vi "Topo & GridSpectr_DriftCorrection_v4.vi"(6 "Internal use":string, 7 "Grid param":T2 {"height (m)" format="%#_6p"; "width (m)" format="%#_6p"; "center Y (m)" format="%#_6p"; "center X (m)" format="%#_6p"}, 8 "Error in (no error)":errorcluster, 9 "Points Y/Index Y":i32, 10 "Points X/Index X":i32, 11 "Method":enum16{"init", "run", "end"}(ring)=enum."end") -> (0 "Error out":errorcluster)   [LabVIEW 2014]
doc: "Example of a measurement VI to be used in the \"Experiments on a Grid\" tool as external VI.\n\nThis example measure the topography and spectroscopy data. The spectroscopy measurements are taken on a subgrid. The data are saved to a sxm and a binary file.\n\n- Nanonis Programming Interface -"
uses:
  <userlib>/Nanonis Prog Interface V5/Nanonis Prog Interface.lvlib
panel:
  in  "STS current step":dbl format="%#_6p"
  in  "tip Speed (m/s)":sgl=3e-09 format="%.2p"
  in  "Drift Correction 2":T1
  out "X drift":i32
  out "Y drift":i32
  out "Queue Steps":i32=40
  in  "StepsBack":i32=40
  in  "Channel index (0-23)":u8=14
  in  "File name":string="10_mol_chain"
  in  "STS Current":dbl=1e-11 format="%#_6p"
  in  "Imaging Current":dbl=1e-10 format="%#_6p"
  in  "zdrift \nDuration (s)":dbl
  in  "Correct z drift":bool
  out "Status":string="init"
  in  "Drift correction Pixels":i32=256 caption="Pixels for drift correction"
  out "Y Offset":dbl
  out "X Offset":dbl
  out "Points taken":dbl
  in  "Drift Correction every":i32=34
  in  "Y subgrid spacing":u16=1
  in  "X subgrid spacing":u16=1
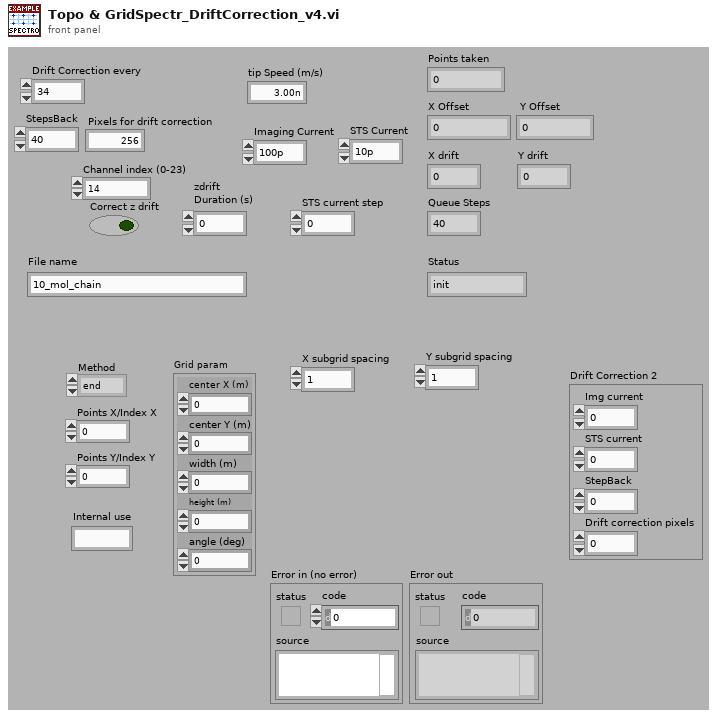
[diagram p1: front panel]
types:
  T1 = cluster{"Img current":dbl, "STS current":dbl, "StepBack":dbl, "Drift correction pixels":dbl}
  T2 = cluster{"center X (m)":sgl, "center Y (m)":sgl, "width (m)":sgl, "height (m)":sgl, "angle (deg)":sgl}
  T3 = cluster{"center X":sgl, "center Y":sgl, "angle":sgl, "width":sgl, "height":sgl, "# pixels":i32, "# lines":i32}
  T4 = cluster{"Name":string, "Calibration":sgl, "Offset":sgl, "Channel index":i32}[]
  T5 = cluster{"up/down":bool, "time/line":sgl, "start time":timestamp, "end time":timestamp}
  T6 = cluster{"Z averaging time (s)":sgl, "Z offset (m)":sgl, "Initial settling time (s)":sgl}
  T7 = cluster{"Max. slew rate (V/s)":sgl, "Settling time (s)":sgl, "Integration time (s)":sgl}
  T8 = cluster{"End settling time (s)":sgl, "Z control time (s)":sgl}
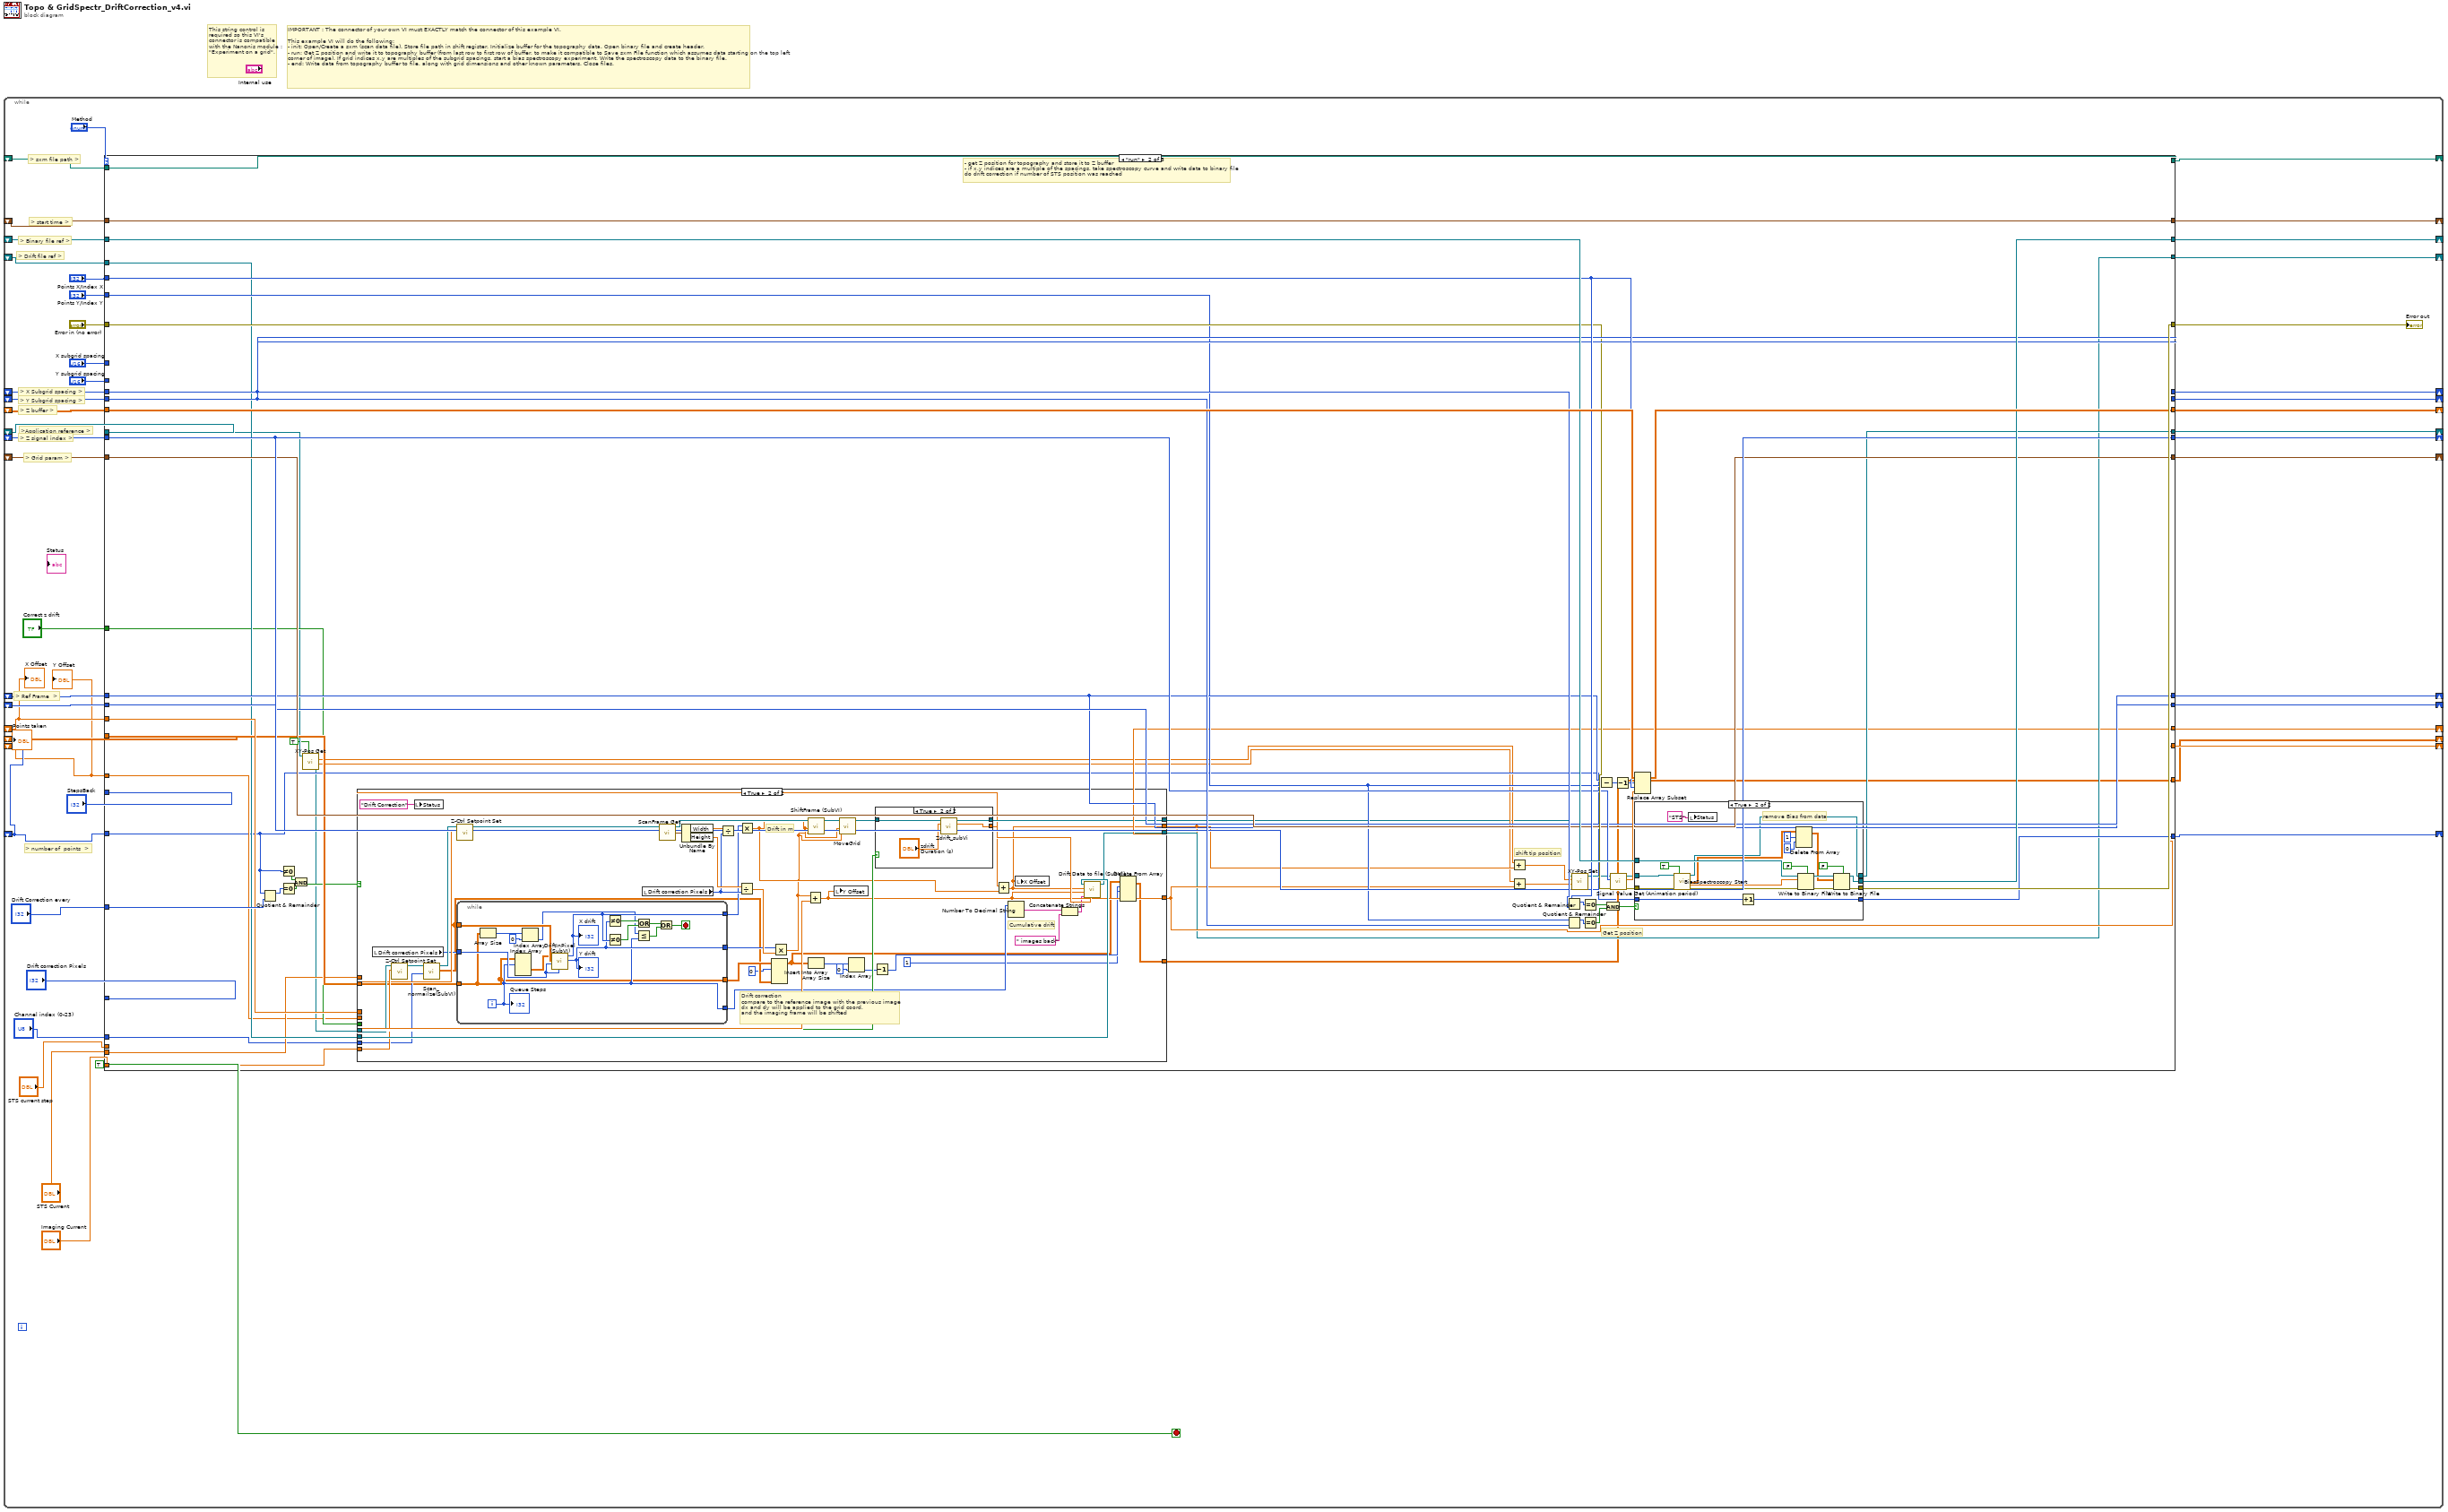
[diagram p0: block diagram]
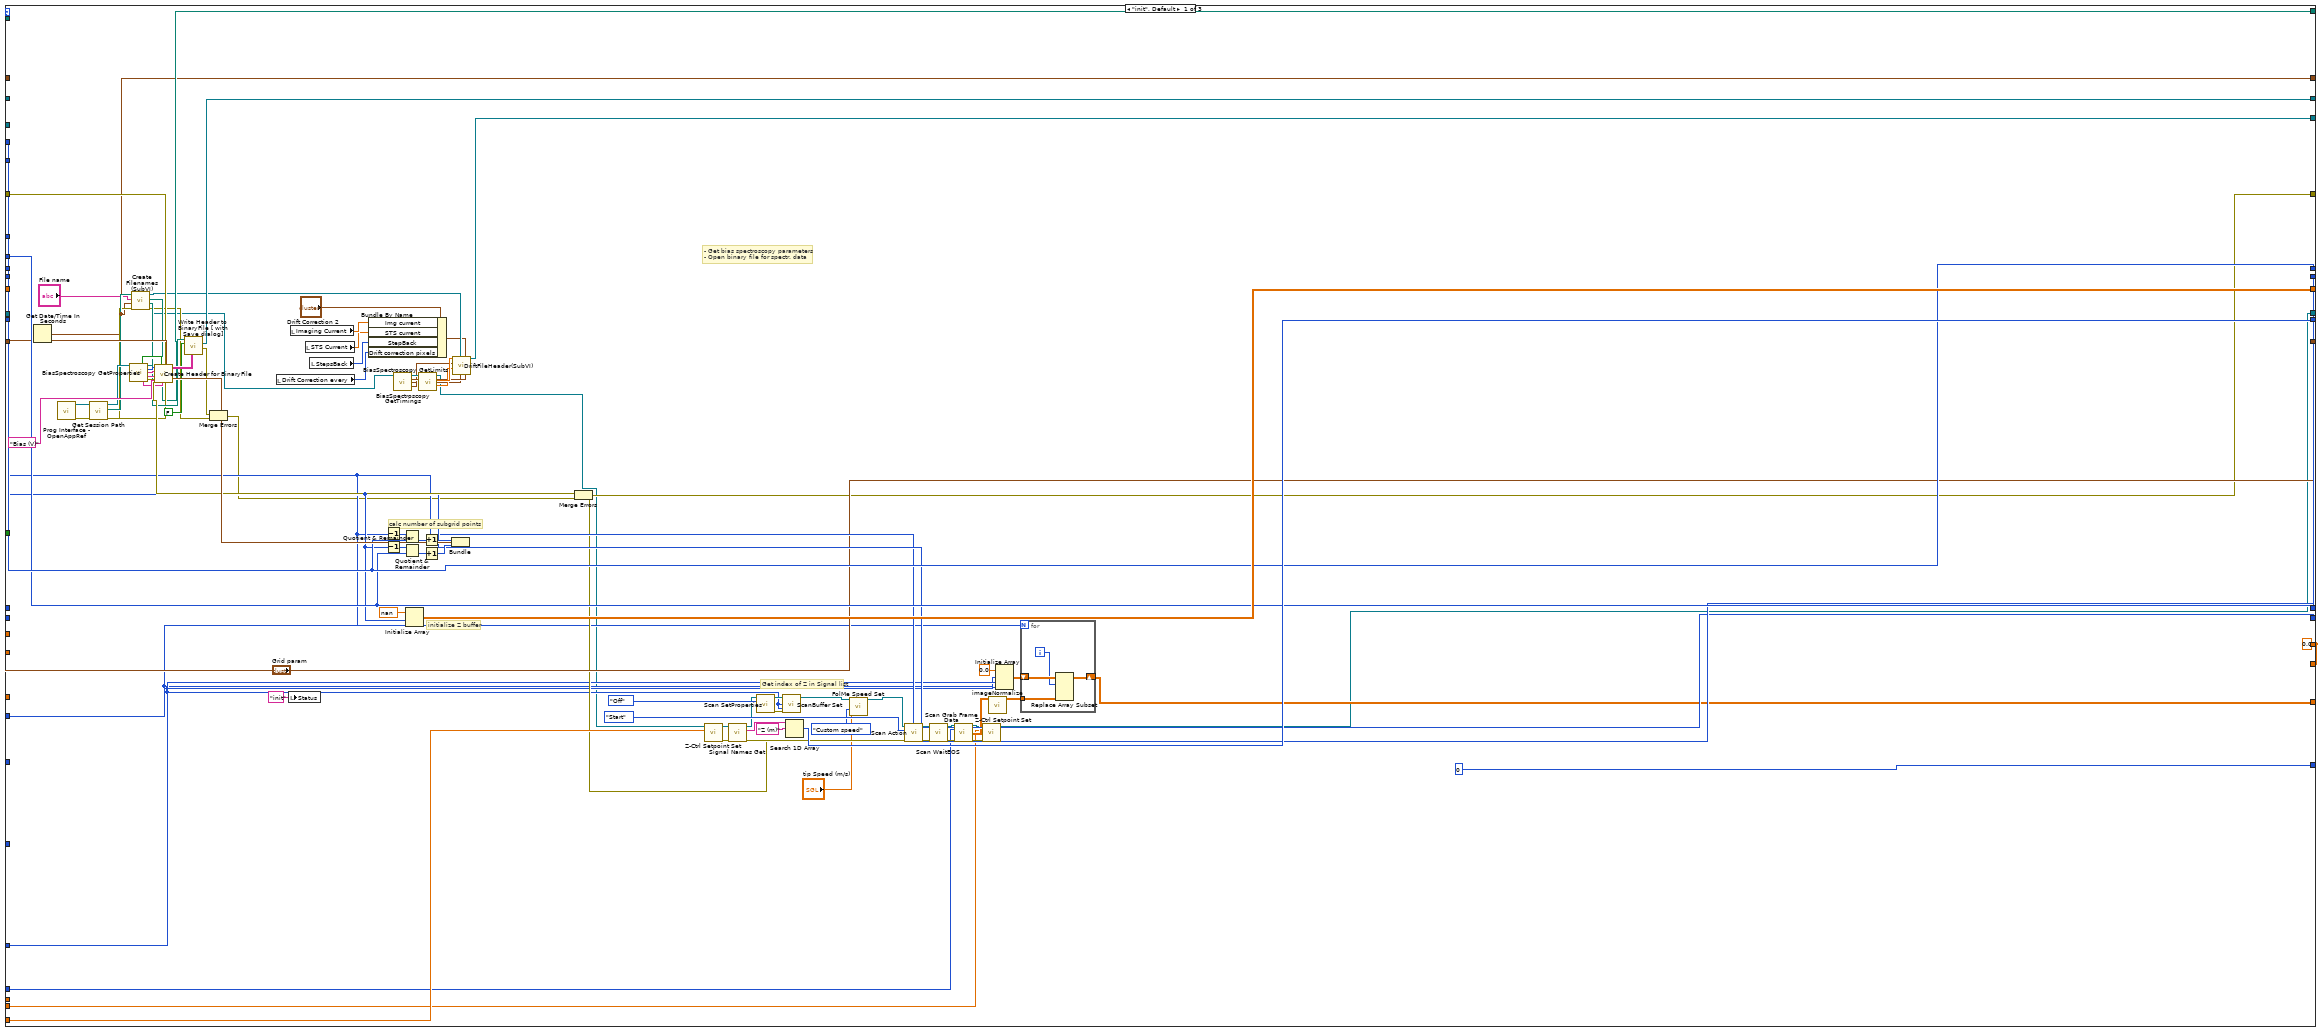
[diagram p2: hidden frame]
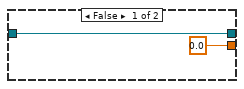
[diagram p4: hidden frame]
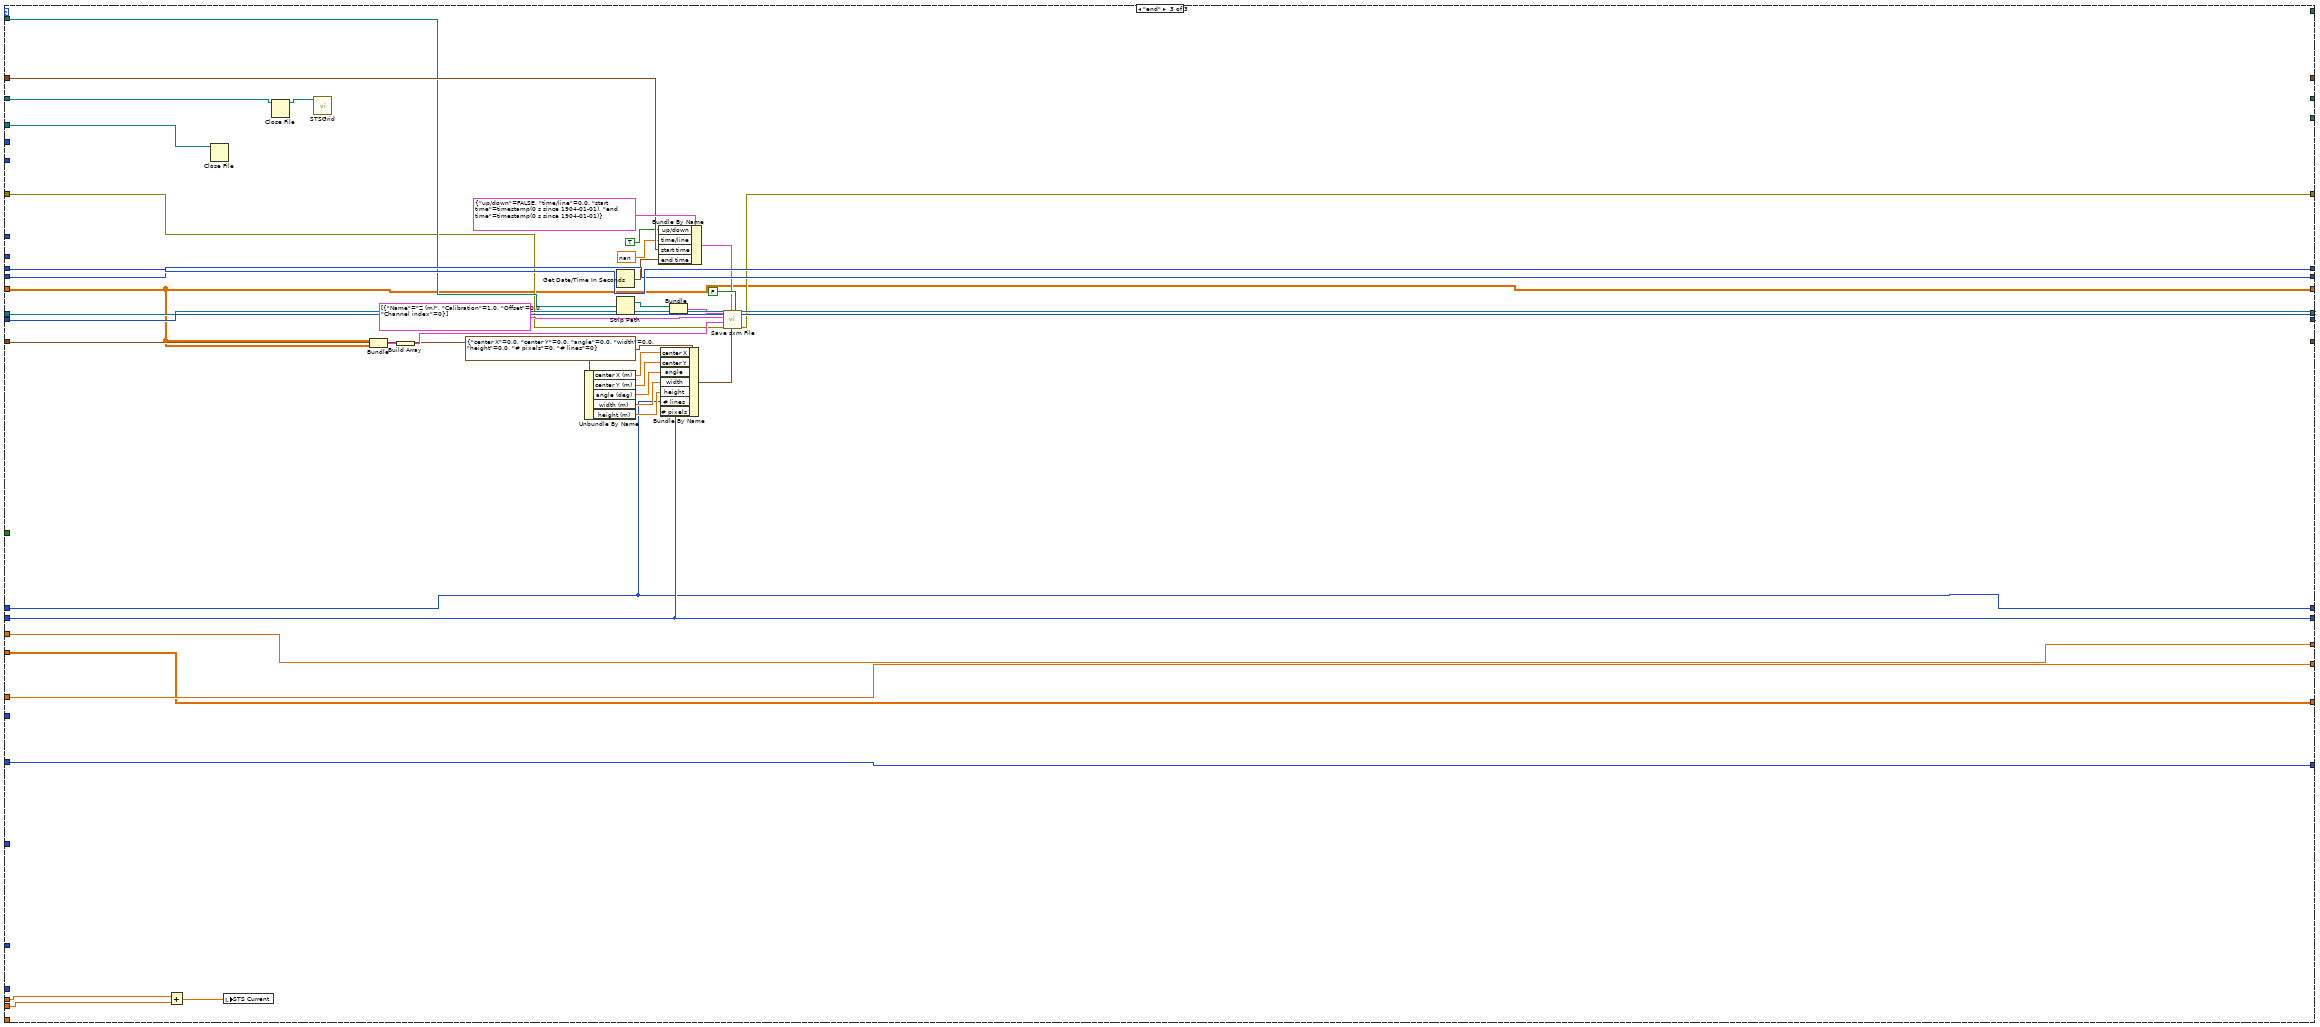
[diagram p6: hidden frame]
diagram:
  # "This string control is required so this VI's connector is compatible with the Nanonis module : \"Experiment on a grid\"."
  # "IMPORTANT : The connector of your own VI must EXACTLY match the connector of this example VI.\n\nThis example VI will do the following:\n- init: Open/Create a sxm (scan data file). Store file path in shift register. Initialize buffer for the topography data. Open binary file and create header.\n- run: Get Z position and write it to topography buffer (from last row to first row of buffer, to make it compatible to Save sxm File function which assumes data starting on the top left corner of image). If grid indices x,y are multiples of the subgrid spacings, start a bias spectroscopy experiment. Write the spectroscopy data to the binary file.\n- end: Write data from topography buffer to file, along with grid dimensions and other known parameters. Close files."
  n1 = while {
    shift-right: [w23] -> _
    shift-left: _ -> [w46]
    shift-right: [w41] -> _
    shift-left: _ -> [w40]
    shift-right: [w38] -> _
    shift-left: _ -> [w39]
    shift-right: [w37] -> _
    shift-left: _ -> [w36]
    shift-right: [w30] -> _
    shift-left: _ -> [w32]
    shift-right: [w31] -> _
    shift-left: _ -> [w33]
    shift-right: [w29] -> _
    shift-left: _ -> [w28]
    shift-right: [w27] -> _
    shift-left: _ -> [w26]
    shift-right: [w25] -> _
    shift-left: _ -> [w24]
    shift-right: [w22] -> _
    shift-left: _ -> [w21]
    shift-right: [w20] -> _
    shift-left: _ -> [w19]
    shift-right: [w18] -> _
    shift-left: _ -> [w11]
    shift-right: [w17] -> _
    shift-left: _ -> [w10]
    shift-right: [w16] -> _
    shift-left: _ -> [w13]
    shift-right: [w15] -> _
    shift-left: _ -> [w12]
    shift-right: [w8] -> _
    shift-left: _ -> [w7]
    stop <- TRUE stop-if-true
    # "> Drift file ref >"
    # "> number of  points  >"
    # "> Ref Frame  >"
    # "> Grid param >"
    # "> start time >"
    # ">Application reference >"
    # "> Y Subgrid spacing >"
    # "> X Subgrid spacing >"
    # "> Z signal index >"
    # "> Binary file ref >"
    # "> Z buffer >"
    # "> sxm file path >"
    n2 = case shown="\"run\"" "Method" {
      tunnel: [w82 w196 _] -> w23
      tunnel: w46 -> [_ w196 w324]
      tunnel: "Error in (no error)" -> [w84 w182 w317]
      tunnel: [w93 w195 w316] -> w44
      tunnel: "Points X/Index X" -> [w113 w190 _]
      tunnel: "Points Y/Index Y" -> [w114 w174 _]
      tunnel: [w137 w193 w305] -> w41
      tunnel: w40 -> [_ w194 w305]
      tunnel: w39 -> [_ w192 w294]
      tunnel: [w129 w191 _] -> w38
      tunnel: [w127 w180 w333] -> w37
      tunnel: w36 -> [_ w180 w333]
      tunnel: "X subgrid spacing" -> [w126 _ _]
      tunnel: "Y subgrid spacing" -> [w125 _ _]
      tunnel: w33 -> [_ w184 w332]
      tunnel: w32 -> [_ w183 w331]
      tunnel: [w126 w184 w332] -> w31
      tunnel: [w125 w183 w331] -> w30
      tunnel: [w55 w166 w330] -> w29
      tunnel: w28 -> [_ w147 w330]
      tunnel: ["Grid param" w177 _] -> w27
      tunnel: w26 -> [_ w177 w315]
      tunnel: [w81 w178 _] -> w25
      tunnel: w24 -> [_ w178 w325]
      tunnel: [w114 w175 w306] -> w22
      tunnel: w21 -> [_ w175 w306]
      tunnel: [w113 w176 w307] -> w20
      tunnel: w19 -> [_ w176 w307]
      tunnel: [w104 w156 w304] -> w18
      tunnel: [w104 w161 w302] -> w17
      tunnel: [w76 w153 w298] -> w16
      tunnel: [0 w171 w303] -> w15
      tunnel: w12 -> [_ w150 w303]
      tunnel: "Drift Correction every" -> [_ w169 _]
      tunnel: w13 -> [_ w160 w298]
      tunnel: w11 -> [_ w167 w304]
      tunnel: w10 -> [_ w151 w302]
      tunnel: "Drift correction Pixels" -> [w75 _ _]
      tunnel: [w71 w158 _] -> w8
      tunnel: w7 -> [_ w159 w299]
      tunnel: "Correct z drift" -> [_ w157 _]
      tunnel: "Imaging Current" -> [w94 w155 _]
      tunnel: "STS Current" -> [w89 w154 w295]
      tunnel: "Channel index (0-23)" -> [w79 w152 _]
      tunnel: "StepsBack" -> [w74 _ _]
      tunnel: "STS current step" -> [_ _ w297]
      frame "init", Default {
        w104 = 0.0
        # "- Get bias spectroscopy parameters\n- Open binary file for spectr. data"
        # "initialize Z buffer"
        # "calc number of subgrid points"
        # "Get index of Z in Signal list"
        n3 = Get Date/Time In Seconds() -> (seconds since 1Jan1904=w81:timestamp)
        n4 = call <userlib>:"Prog Interface - OpenAppRef.vi"("Error in (no error)"=w84) -> ("Error out"=w86:errorcluster, "Application reference"=w88:refnum<vi>)  [unwired: 5 in]
        n5 = call <userlib>:"Get Session Path.vi"("error in (no error)"=w86, "Application ref in"=w88) -> ("error out"=w83:errorcluster, "Session path"=w85:path, "Application ref out"=w87:refnum<vi>)  [unwired: 7 in]
        n6 = call <userlib>:"BiasSpectroscopy GetProperties.vi"("Application ref in"=w87) -> ("Backward sweep"=w133:bool, "Application ref out"=w54:refnum<vi>, "Number of points"=w116:i32, "Channels"=w115:string[], "Parameters"=w131:string[], "Fixed parameters"=w118:string[], "Error out"=w130:errorcluster)  [unwired: 6 in, 2 out]
        n7 = call "Create Filenames (SubVI).vi"("error in (no error)"=w83, "seconds since 1Jan1904"=w81, "File name"="File name", "Session path"=w85) -> ("error out"=w56:errorcluster, "binFilePath"=w97:path, "topoFilePath"=w82:path, "Drift File out"=w72:refnum<file>)  [unwired: 4 in]
        n8 = local read "Drift Correction every"() -> (w66:i32)
        n9 = local write "Status"("init" ("Status")) -> ()
        n10 = local read "Imaging Current"() -> (w68:dbl)
        n11 = local read "STS Current"() -> (w67:dbl)
        n12 = local read "StepsBack"() -> (w65:i32)
        n13 = Bundle By Name(cluster="Drift Correction 2", "Img current"=w68, "STS current"=w67, "StepBack"=w65, "Drift correction pixels"=w66) -> (w69:T1)
        n14 = Decrement(x=w113) -> (x-1=w124:i32)
        n15 = Decrement(x=w114) -> (x-1=w123:i32)
        n16 = call <userlib>:"BiasSpectroscopy GetTimings.vi"("Application ref in"=w54) -> ("Application ref out"=w64:refnum<vi>, "Initialization"=w61:T6, "Sweep Timing"=w59:T7, "End of Sweep"=w60:T8)  [unwired: 10 in, 1 out]
        n17 = Quotient & Remainder(x=w124, y=w126) -> (floor(x/y)=w122:i32)  [unwired: 1 out]
        n18 = Quotient & Remainder(x=w123, y=w125) -> (floor(x/y)=w121:i32)  [unwired: 1 out]
        n19 = Initialize Array(sgl nan ("element"), w114, w113) -> (w137:sgl[][])
        n20 = call <userlib>:"BiasSpectroscopy GetLimits.vi"("Application ref in"=w64) -> ("End value (V)"=w62:sgl, "Start value (V)"=w63:sgl, "Application ref out"=w53:refnum<vi>)  [unwired: 5 in, 1 out]
        n21 = Increment(x=w122) -> (x+1=w120:i32)
        n22 = Increment(x=w121) -> (x+1=w119:i32)
        n23 = Bundle(w120, w119) -> (w132:cluster{i32, i32})  [unwired: 1 in]
        n24 = call <userlib>:"Create Header for BinaryFile.vi"("Grid points"=w132, "Grid param"="Grid param", "Fixed parameters"=w118, "Backward sweep"=w133, "Sweep signal"="Bias (V)" ("Sweep Signal"), "Parameters"=w131, "Channels"=w115, "Points per sweep"=w116) -> ("Header (fixed attributes)"=w135:string[][])  [unwired: 3 in]
        n25 = call <userlib>:"Write Header to BinaryFile [ with Save dialog].vi"("Fixed Attributes"=w135, "Show Dialog? (T)"=FALSE, "Filename"=w97) -> ("Error out"=w57:errorcluster, "File ref"=w129:refnum<file>)  [unwired: 5 in, 2 out]
        n26 = Merge Errors(w57, w56) -> (w58:errorcluster)
        n27 = call "DriftFileHeader(SubVI).vi"("Initialization"=w61, "Drift Correction"=w69, "Sweep Timing"=w59, "Byte Stream File in"=w72, "End value (V)"=w62, "End of Sweep"=w60, "Start value (V)"=w63) -> ("Byte Stream File out"=w71:refnum<file>)  [unwired: 4 in]
        n28 = Merge Errors(w130, w58) -> (w93:errorcluster)
        n29 = call <userlib>:"Z-Ctrl Setpoint Set.vi"("error in (no error)"=w93, "Z Controller setpoint"=w94, "Application ref in"=w53) -> ("error out"=w92:errorcluster, "Application ref out"=w95:refnum<vi>)  [unwired: 7 in]
        n30 = call <userlib>:"Signal Names Get.vi"("error in (no error)"=w92, "Application ref in"=w95) -> ("error out"=w105:errorcluster, "Signals Names"=w117:string[], "Application ref out"=w100:refnum<vi>)  [unwired: 5 in]
        n31 = call <userlib>:"Scan SetProperties.vi"("Application ref in"=w100, "Continuous scan"=enum16{"No change", "On", "Off"}."Off") -> ("Application ref out"=w102:refnum<vi>, "Error out"=w101:errorcluster)  [unwired: 12 in]
        n32 = call <userlib>:"ScanBuffer Set.vi"("Application ref in"=w102, "Pixels"=w75, "Lines"=w75, "error in (no error)"=w101) -> ("Application ref out"=w52:refnum<vi>)  [unwired: 10 in, 1 out]
        n33 = Search 1D Array(1D array=w117, element="Z (m)") -> (index of element=w127:i32)  [unwired: 1 in]
        n34 = call <userlib>:"FolMe Speed Set.vi"("Speed Setting (Custom)"=enum32{"Scan speed", "Custom speed"}."Custom speed", "Speed (m/s)"="tip Speed (m/s)", "Application ref in"=w52) -> ("Application ref out"=w51:refnum<vi>)  [unwired: 5 in, 1 out]
        n35 = call <userlib>:"Scan Action.vi"("error in (no error)"=w105, "Scan action (Start)"=enum16{"Start", "Stop", "Pause", "Resume"}."Start", "Application ref in"=w51) -> ("error out"=w111:errorcluster, "Application ref out"=w110:refnum<vi>)  [unwired: 6 in]
        n36 = call <userlib>:"Scan WaitEOS.vi"("error in (no error)"=w111, "Application ref in"=w110) -> ("error out"=w108:errorcluster, "Application ref out"=w109:refnum<vi>)  [unwired: 5 in, 2 out]
        n37 = call <userlib>:"Scan Grab Frame Data.vi"("Application ref in"=w109, "Channel index (0-23)"=w79, "error in (no error)"=w108) -> ("Application ref out"=w91:refnum<vi>, "Scan frame data"=w96:sgl[][], "error out"=w90:errorcluster)  [unwired: 8 in, 2 out]
        n38 = call <userlib>:"Z-Ctrl Setpoint Set.vi"("error in (no error)"=w90, "Z Controller setpoint"=w89, "Application ref in"=w91) -> ("Application ref out"=w55:refnum<vi>)  [unwired: 7 in, 1 out]
        n39 = call "imageNormalize.vi"("Data"=w96) -> ("Array"=w73:dbl[][])  [unwired: 10 in]
        n40 = Initialize Array(0.0 ("element"), w74, w75, w75) -> (w77:dbl[][][])
        n41 = for {
          N: w74 -> [_]
          tunnel: w73 -> [w140]
          shift-right: [w139] -> w76
          shift-left: w77 -> [w141]
          i -> [w138]
          n42 = Replace Array Subset(array=w141, new element=w140, index (dim 0)=w138) -> (w139:dbl[][][])  [unwired: 2 in]
        }
      }
      frame "run" {
        # "shift tip position"
        # "Get Z position"
        # "- get Z position for topography and store it to Z buffer\n- if x,y indices are a multiple of the spacings, take spectroscopy curve and write data to binary file\ndo drift correction if number of STS position was reached"
        n43 = Quotient & Remainder(x=w150, y=w169) -> (x-y*floor(x/y)=w170:i32)  [unwired: 1 out]
        n44 = Not Equal To 0?(x=w150) -> (x != 0?=w148:bool)
        n45 = Equal To 0?(x=w170) -> (x = 0?=w168:bool)
        n46 = And(x=w148, y=w168) -> (x .and. y?=w149:bool)
        n47 = call <userlib>:"XY-Pos Get.vi"("Wait for newest data (F=False)"=TRUE, "Application ref in"=w147) -> ("Y (m)"=w143:sgl, "X (m)"=w144:sgl, "Application ref out"=w146:refnum<vi>)  [unwired: 5 in, 1 out]
        n48 = case shown="True" w149 {
          tunnel: w146 -> [w201 w232]
          tunnel: [w201 w238] -> w142
          tunnel: w160 -> [w198 w220]
          tunnel: [w200 w234] -> w156
          tunnel: [w199 w233] -> w161
          tunnel: w167 -> [w200 w236]
          tunnel: w151 -> [w199 w237]
          tunnel: [w198 w212] -> w153
          tunnel: w159 -> [w197 w241]
          tunnel: [w197 w240] -> w158
          tunnel: w157 -> [_ w235]
          tunnel: w155 -> [_ w231]
          tunnel: w154 -> [_ w229]
          tunnel: w152 -> [_ w224]
          frame False {
          }
          frame True {
            # "Cumulative drift"
            # "Drift in m"
            # "Drift correction \ncompare to the reference image with the previous image \ndx and dy will be applied to the grid coord, \nand the imaging frame will be shifted"
            n49 = local read "Drift correction Pixels"() -> (w223:i32)
            n50 = call <userlib>:"Z-Ctrl Setpoint Set.vi"("Z Controller setpoint"=w231, "Application ref in"=w232) -> ("Application ref out"=w228:refnum<vi>)  [unwired: 8 in, 1 out]
            n51 = local write "Status"("Drift Correction" ("Status")) -> ()
            n52 = call "Scan_normailze(SubVI).vi"("Channel index (0-23)"=w224, "Application in"=w228) -> ("Array"=w214:dbl[][], "Application out"=w230:refnum<vi>)  [unwired: 7 in, 1 out]
            n53 = call <userlib>:"Z-Ctrl Setpoint Set.vi"("Z Controller setpoint"=w229, "Application ref in"=w230) -> ("Application ref out"=w226:refnum<vi>)  [unwired: 8 in, 1 out]
            n54 = while {
              tunnel: w223 -> [w260]
              tunnel: w214 -> [w259]
              tunnel: w220 -> [w249]
              tunnel: [w258] -> w222
              tunnel: [w257] -> w221
              tunnel: [w253] -> w219
              tunnel: [w249] -> w215
              i -> [w253]
              stop <- w255 stop-if-true
              n55 = Array Size(array=w249) -> (size(s)=w252:i32[])
              n56 = Index Array(array=w249, index (dim 0)=w253) -> (element=w248:dbl[][])  [unwired: 2 in]
              n57 = Index Array(array=w252, index=0) -> (element=w250:i32)
              n58 = call "DriftInPixel (SubVI).vi"(6:w260, 9:w260, "New image"=w259, "Ref image"=w248) -> ("Y drift"=w257:i32, "X drift"=w258:i32)  [unwired: 5 in, 1 out]
              "Y drift" <- w257
              "X drift" <- w258
              n59 = Not Equal To 0?(x=w257) -> (x != 0?=w262:bool)
              n60 = Not Equal To 0?(x=w258) -> (x != 0?=w261:bool)
              n61 = Or(x=w262, y=w261) -> (x .or. y?=w256:bool)
              n62 = Less Or Equal?(x=w250, y=w253) -> (x <= y?=w254:bool)
              n63 = Or(x=w256, y=w254) -> (x .or. y?=w255:bool)
              "Queue Steps" <- w253
            }
            n64 = local read "Drift correction Pixels"() -> (w225:i32)
            n65 = call <userlib>:"ScanFrame Get.vi"("Application ref in"=w226) -> ("Application ref out"=w227:refnum<vi>, "Size (m)"=w246:cluster{"Width":sgl, "Height":sgl})  [unwired: 10 in, 3 out]
            n66 = Unbundle By Name(w246) -> ("Width"=w245:sgl, "Height"=w247:sgl)
            n67 = Divide(x=w245, y=w225) -> (x/y=w244:sgl)
            n68 = Divide(x=w247, y=w225) -> (x/y=w243:sgl)
            n69 = Multiply(x=w222, y=w244) -> (x*y=w203:sgl)
            n70 = Insert Into Array(array=w215, index (dim 0)=0 ("index (page)"), new element=w214) -> (w211:dbl[][][])  [unwired: 2 in]
            n71 = Multiply(x=w221, y=w243) -> (x*y=w202:sgl)
            n72 = Add(x=w202, y=w237) -> (x+y=w233:dbl)
            n73 = call "ShiftFrame (SubVI).vi"("Y shift"=w202, "X shift"=w203, "Application in"=w227) -> ("Application out"=w205:refnum<vi>)  [unwired: 8 in]
            n74 = Array Size(array=w211) -> (size(s)=w210:i32[])
            n75 = local write "Y Offset"(w233) -> ()
            n76 = call "MoveGrid.vi"("y"=w202, "x"=w203, "Application ref in"=w205) -> ("Application ref out"=w204:refnum<vi>)  [unwired: 7 in, 1 out]
            n77 = Index Array(array=w210, index=0) -> (element=w208:i32)
            n78 = Decrement(x=w208) -> (x-1=w207:i32)
            n79 = case shown="True" w235 {
              tunnel: [0.0 ("z drift") w268] -> w239
              tunnel: w204 -> [w263 w267]
              tunnel: [w263 w266] -> w238
              frame False {
              }
              frame True {
                n80 = call "Zdrift_subVi.vi"("Duration"="zdrift \nDuration (s)", "Application in"=w267) -> ("z drift"=w268:dbl, "Application out"=w266:refnum<vi>)  [unwired: 7 in, 1 out]
              }
            }
            n81 = Add(x=w236, y=w203) -> (x+y=w234:dbl)
            n82 = Number To Decimal String(number=w219) -> (decimal integer string=w218:string)  [unwired: 1 in]
            n83 = local write "X Offset"(w234) -> ()
            n84 = Concatenate Strings(w218, " images back" ("string")) -> (w217:string)
            n85 = call "Drift Data to file (SubVI).vi"("z drift"=w239, "Comment"=w217, "y Drift"=w233, "X drift"=w234, "Byte Stream File in"=w241) -> ("Byte Stream File out"=w240:refnum<file>)  [unwired: 6 in]
            n86 = Delete From Array(array=w211, length=1, index (dim 0)=w207) -> (array with subset deleted=w212:dbl[][][])  [unwired: 2 in, 1 out]
          }
        }
        n87 = Add(x=w144, y=w156) -> (x+y=w163:dbl)
        n88 = Add(x=w143, y=w161) -> (x+y=w162:dbl)
        n89 = Quotient & Remainder(x=w190, y=w184) -> (x-y*floor(x/y)=w189:i32)  [unwired: 1 out]
        n90 = Quotient & Remainder(x=w174, y=w183) -> (x-y*floor(x/y)=w188:i32)  [unwired: 1 out]
        n91 = call <userlib>:"XY-Pos Set.vi"("Y (m)"=w162, "X (m)"=w163, "Application ref in"=w142) -> ("Application ref out"=w164:refnum<vi>)  [unwired: 5 in, 1 out]
        n92 = Equal To 0?(x=w189) -> (x = 0?=w187:bool)
        n93 = Equal To 0?(x=w188) -> (x = 0?=w186:bool)
        n94 = Subtract(x=w175, y=w174) -> (x-y=w173:i32)
        n95 = And(x=w187, y=w186) -> (x .and. y?=w185:bool)
        n96 = call <userlib>:"Signal Value Get (Animation period).vi"("error in (no error)"=w182, "Signal index (0-47)"=w180, "Application ref in"=w164) -> ("error out"=w181:errorcluster, "Signal value"=w179:sgl, "Application ref out"=w165:refnum<vi>)  [unwired: 5 in]
        n97 = Decrement(x=w173) -> (x-1=w172:i32)
        n98 = Replace Array Subset(array=w194, new element=w179, index (row)=w172, index (col)=w190) -> (w193:sgl[][])
        n99 = case shown="True" w185 {
          tunnel: [w271 w276] -> w195
          tunnel: w192 -> [w272 w292]
          tunnel: [w272 w290] -> w191
          tunnel: w181 -> [w271 w289]
          tunnel: w165 -> [w270 w281]
          tunnel: [w270 w280] -> w166
          tunnel: [w269 w274] -> w171
          tunnel: w150 -> [w269 w275]
          frame False {
            # "Point indices aren't multiple of subgrid spacing\n=> no spectroscopy at this point"
          }
          frame True {
            # "remove Bias from data"
            n100 = call <userlib>:"BiasSpectroscopy Start.vi"("Application ref in"=w281, "Get data (F)"=TRUE ("Get Data (F)"), "Error in (no error)"=w289) -> ("Application ref out"=w280:refnum<vi>, "Data"=w288:sgl[][], "Parameters"=w287:sgl[], "Error out"=w278:errorcluster)  [unwired: 8 in, 1 out]
            n101 = local write "Status"("STS" ("Status")) -> ()
            n102 = Increment(x=w275) -> (x+1=w274:i32)
            n103 = Delete From Array(array=w288, length=1, index (row)=0 ("index")) -> (array with subset deleted=w286:sgl[][])  [unwired: 1 in, 1 out]
            n104 = Write to Binary File(file (use dialog)=w292, data=w287, error in=w278, 5:FALSE ("prepend array or string size? (T)")) -> (refnum out=w291:refnum<file>, error out=w277:errorcluster)  [unwired: 2 in, 1 out]
            n105 = Write to Binary File(file (use dialog)=w291, data=w286, error in=w277, 5:FALSE ("prepend array or string size? (T)")) -> (refnum out=w290:refnum<file>, error out=w276:errorcluster)  [unwired: 2 in, 1 out]
          }
        }
      }
      frame "end" {
        n106 = Add(x=w297, y=w295) -> (x+y=w296:dbl)
        n107 = Close File(refnum=w299) -> ()  [unwired: 1 in, 2 out]
        n108 = local write "STS Current"(w296) -> ()
        n109 = Close File(refnum=w294) -> (path=w293:path)  [unwired: 1 in, 1 out]
        n110 = call "STSGrid.vi"("Binary Spectroscopy File"=w293) -> ()  [unwired: 11 in]
        n111 = Bundle(w305, w305) -> (w329:cluster{sgl[][], sgl[][]})  [unwired: 1 in]
        n112 = Build Array(w329) -> (w328:cluster{sgl[][], sgl[][]}[])
        n113 = Unbundle By Name(w315) -> ("center X (m)"=w313:sgl, "center Y (m)"=w312:sgl, "angle (deg)"=w311:sgl, "width (m)"=w310:sgl, "height (m)"=w309:sgl)
        n114 = Get Date/Time In Seconds() -> (seconds since 1Jan1904=w301:timestamp)
        n115 = Strip Path(path=w324) -> (stripped path=w320:path, name=w319:string)
        n116 = Bundle By Name(cluster=T5 {"up/down"=FALSE, "time/line"=0.0, "start time"=timestamp(0 s since 1904-01-01), "end time"=timestamp(0 s since 1904-01-01)} ("Scan param"), "up/down"=TRUE, "time/line"=sgl nan ("input 7"), "start time"=w325, "end time"=w301) -> (w323:T5)
        n117 = Bundle By Name(cluster=T3 {"center X"=0.0, "center Y"=0.0, "angle"=0.0, "width"=0.0, "height"=0.0, "# pixels"=0, "# lines"=0} ("Scanfield"), "center X"=w313, "center Y"=w312, "angle"=w311, "width"=w310, "height"=w309, "# lines"=w306, "# pixels"=w307) -> (w308:T3)
        n118 = Bundle("stripped path"=w320, "name"=w319) -> (w318:cluster{"stripped path":path, "name":string})  [unwired: 1 in]
        n119 = call <userlib>:"Save sxm File.vi"("Auto file naming? (T)"=FALSE, "Scanfield"=w308, "Scan param"=w323, "error in (no error)"=w317, "Channels data"=w328, "Channels config"=T4 [{"Name"="Z (m)", "Calibration"=1.0, "Offset"=0.0, "Channel index"=0}], "Filename control"=w318) -> ("error out"=w316:errorcluster)  [unwired: 2 in, 2 out]
      }
    }
    "Error out" <- w44
    "Points taken" <- w12
    "X Offset" <- w11
    "Y Offset" <- w10
  }
